vi "UploadAcquisitions.vi"(8 "error in (no error)":errorcluster, 10 "Acquisitions":T1, 11 "ByteGSAPIBase in":refnum<class "ByteGSAPIBase.lvclass">) -> (0 "error out":errorcluster, 3 "ByteGSAPIBase out":refnum<class "ByteGSAPIBase.lvclass">)   [LabVIEW 2019, in "ByteGSWebAPI.lvlib" / "ByteGSAPIBase.lvclass"]
uses:
  ByteGSAPIBase.lvclass
  acquisitions.ctl
  ByteGSAPIBase.lvclass/ByteGSAPIBase.ctl
  <vilib>/Bytelabs/ByteREST/ByteRESTClass/ByteRESTBase/RESTBase.lvclass
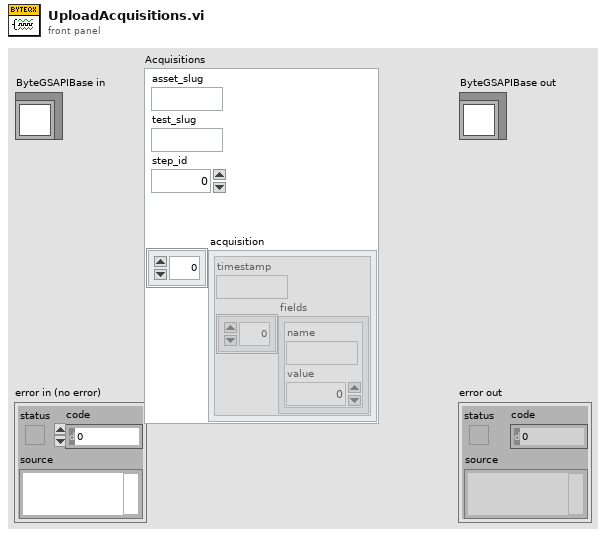
[diagram p1: front panel]
types:
  T1 = typedef "ByteGSWebAPI.lvlib/ByteGSAPIBase.lvclass/acquisitions.ctl" = cluster{"asset_slug":string, "test_slug":string, "step_id":i32, "acquisition":cluster{"timestamp":string, "fields":cluster{"name":string, "value":dbl}[]}[]}
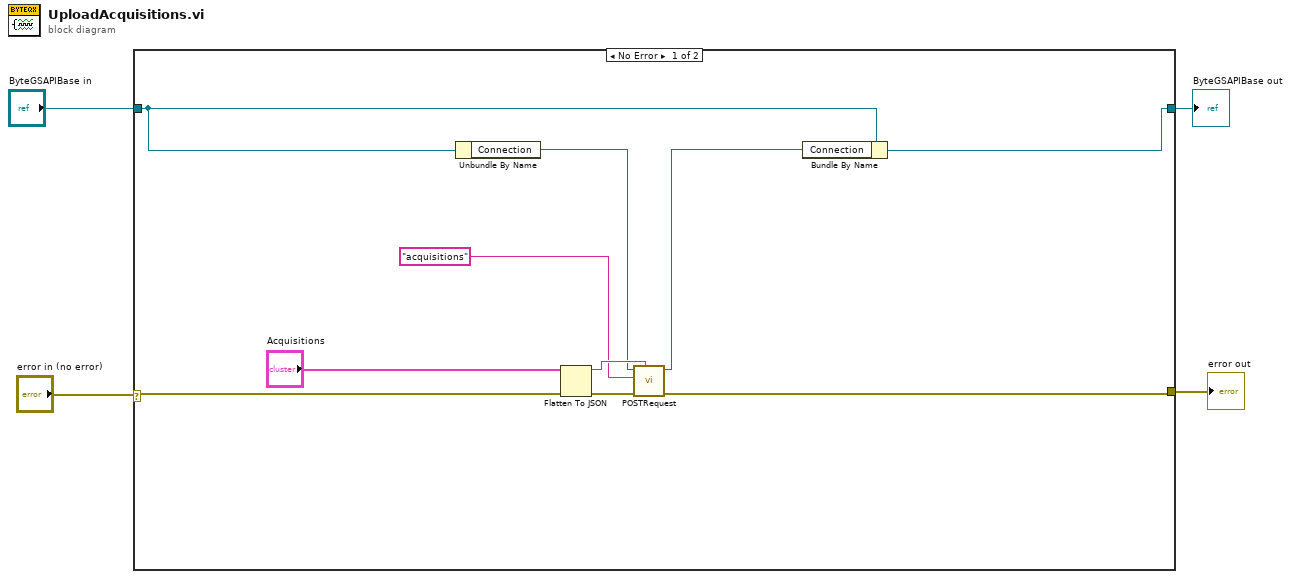
[diagram p0: block diagram]
diagram:
  n1 = case shown="No Error" "error in (no error)" {
    selector: "error in (no error)" -> [w8 w16]
    tunnel: [w6 w16] -> w3
    tunnel: [w13 w15] -> w1
    tunnel: "ByteGSAPIBase in" -> [w14 w15]
    frame No Error {
      n2 = Unbundle By Name(w14) -> ("Connection"=w10:refnum<class "RESTBase.lvclass">)
      n3 = Flatten To JSON(anything="Acquisitions", error in (no error)=w8) -> (JSON string=w12:string, 11:w11:errorcluster)  [unwired: 1 in]
      n4 = call-dynamic "POSTRequest.vi"("Body in"=w12, "error in (no error)"=w11, "Request"="acquisitions", "ByteRESTBase in"=w10) -> ("error out"=w6:errorcluster, "ByteRESTBase out"=w9:refnum<class "RESTBase.lvclass">)  [unwired: 4 in, 2 out]
      n5 = Bundle By Name(cluster=w14, "Connection"=w9) -> (w13:refnum<class "ByteGSAPIBase.lvclass">)
    }
    frame Error {
    }
  }
  "error out" <- w3
  "ByteGSAPIBase out" <- w1
